vi "DFD IIR Notch Peak Design by BW.vi"(6 "fs [Hz]":dbl=1.0 format="%.2f", 7 "filter type":enum16{"Notch", "Peak"}(ring), 8 "error in (no error)":errorcluster, 9 "Ab [dB]":dbl=3.010299956639812 format="%#.6g", 10 "Df [Hz]":dbl=0.02 format="%.2f", 11 "f0 [Hz]":dbl=0.1 format="%.2f") -> (0 "error out":errorcluster, 3 "filter out":T1={"mSRate_Fs"=1.0, "mSRate_Version"="2.0", "mSRate_Comments"="", "mSRate_OrgCoef"={"type"=enum."Undefined", "gain"=1.0, "coef a (k)"=[], "coef b (v)"=[]}, "mSRate_CurCoef"={"type"=enum."Undefined", "gain"=1.0, "coef a (k)"=[], "coef b (v)"=[]}, "mSRate_Quantized?"=FALSE, "mSRate_QCoef"={"type"=enum."Undefined", "gain"=1.0, "coef a (k)"=[], "coef b (v)"=[]}, "mSRate_QSettings"=[], "mSRate_Order"=0, "mSRate_Scaling"={"mSRate_ScaleByPowerOf2?"=FALSE, "mSRate_ScaleType"=enum."No Norm"}} {"mSRate_QSettings"."source" items=["Coef a/k"=0, "Coef b/v"=7, "Input"=1, "Output"=2, "Multiplicand"=3, "Product"=4, "Sum"=5, "Delay"=6, "Gain"=8]})   [LabVIEW 2017, in "NI_DigFilterLicensed.lvlib"]
doc: "Designs a notch or peak filter in which the notch or peak is located at the center frequency. You must manually select the polymorphic instance you want to use."
uses:
  <vilib>/addons/Digital Filter Design/NI_DigFilterLicensed.lvlib
  <vilib>/addons/Digital Filter Design/_Objects.llb/DFD Filter Obj.ctl
  <vilib>/addons/Digital Filter Design/_Objects.llb/DFD Filter Coef.ctl
  <vilib>/addons/Digital Filter Design/_Objects.llb/DFD Filter Structure Type Selector.ctl
  <vilib>/addons/Digital Filter Design/_Objects.llb/dfd_Internal Quantization Settings.ctl
  <vilib>/addons/Digital Filter Design/_Objects.llb/dfd_Internal Quantization Srcs.ctl
  <vilib>/addons/Digital Filter Design/_Objects.llb/DFD Coef Norm Type.ctl
  <vilib>/addons/Digital Filter Design/NI_DigFilter_Design.lvlib
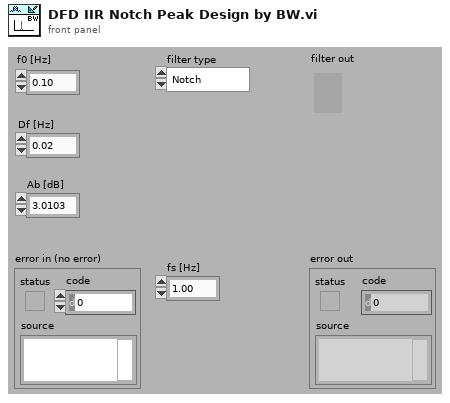
[diagram p1: front panel]
types:
  T1 = typedef "NI_DigFilterLicensed.lvlib/DFD Filter Obj.ctl" = cluster{"mSRate_Fs":dbl, "mSRate_Version":string, "mSRate_Comments":string, "mSRate_OrgCoef":T2, "mSRate_CurCoef":T2, "mSRate_Quantized?":bool, "mSRate_QCoef":T2, "mSRate_QSettings":T4[], "mSRate_Order":i32, "mSRate_Scaling":cluster{"mSRate_ScaleByPowerOf2?":bool, "mSRate_ScaleType":T6}}
  T2 = typedef "NI_DigFilterLicensed.lvlib/DFD Filter Coef.ctl" = cluster{"type":T3, "gain":dbl, "coef a (k)":dbl[], "coef b (v)":dbl[]}
  T3 = typedef "NI_DigFilterLicensed.lvlib/DFD Filter Structure Type Selector.ctl" = enum16{"Undefined", "FIR Direct Form", "FIR Direct Form Transposed", "FIR Symmetric", "FIR Antisymmetric", "IIR Direct Form I", "IIR Direct Form I Transposed", "IIR Direct Form II", "IIR Direct Form II Transposed", "IIR Cascaded Second Order Sections Form I", "IIR Cascaded Second Order Sections Form I Transposed", "IIR Cascaded Second Order Sections Form II", "IIR Cascaded Second Order Sections Form II Transposed", "Lattice Allpass (basic sections)", "Lattice Allpass (one multiplier sections)", "Lattice Allpass (normalized sections)", "Lattice AR (basic sections)", "Lattice AR (one multiplier sections)", "Lattice AR (normalized sections)", "Lattice MA (minimum phase)", "Lattice MA (maximum phase)", "Lattice ARMA (basic sections)", "Lattice ARMA (one multiplier sections)", "Lattice ARMA (normalized sections)"}
  T4 = typedef "NI_DigFilterLicensed.lvlib/dfd_Internal Quantization Settings.ctl" = cluster{"source":T5, "wl":i16, "iwl":i16, "overflow mode":enum16{"Saturation", "Wrap"}, "rounding mode":enum16{"Nearest", "Truncation"}, "signed?":bool}
  T5 = typedef "NI_DigFilterLicensed.lvlib/dfd_Internal Quantization Srcs.ctl" = u16
  T6 = typedef "NI_DigFilterLicensed.lvlib/DFD Coef Norm Type.ctl" = enum16{"No Norm", "Time Domain 1-Norm", "Time Domain 2-Norm", "Time Domain Inf-Norm"}
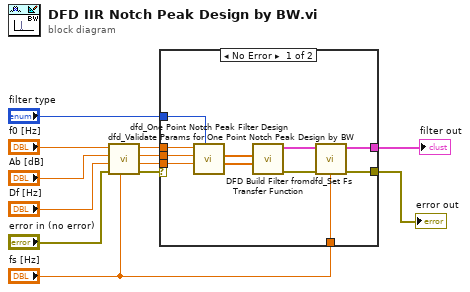
[diagram p0: block diagram]
diagram:
  n1 = call <vilib>:"dfd_Validate Params for One Point Notch Peak Design by BW.vi"("fs [Hz]"="fs [Hz]", "error in (no error)"="error in (no error)", "bandwidth"="Df [Hz]", "Ab [dB]"="Ab [dB]", "f0 [Hz]"="f0 [Hz]") -> ("error out"=w1:errorcluster, "normalized bandwidth"=w2:dbl, "dup Ab [dB]"=w3:dbl, "normalized f0"=w4:dbl)  [unwired: 3 out]
  n2 = case shown="No Error" w1 {
    selector: w1 -> [_ w24]
    tunnel: [w23 w24] -> w12
    tunnel: [w22 _] -> w11
    tunnel: "filter type" -> [w21 _]
    tunnel: w4 -> [w16 _]
    tunnel: w3 -> [w15 _]
    tunnel: w2 -> [w14 _]
    tunnel: "fs [Hz]" -> [w13 _]
    frame No Error {
      n3 = call <vilib>:"dfd_One Point Notch Peak Filter Design.vi"("filter type"=w21, "normalized BW"=w14, "Ab [dB]"=w15, "normalized f0"=w16) -> ("denominator"=w17:dbl[], "numerator"=w18:dbl[])  [unwired: 2 in, 4 out]
      n4 = call <vilib>:"DFD Build Filter from Transfer Function.vi"("denominator"=w17, "numerator"=w18) -> ("error out"=w19:errorcluster, "filter out"=w20:T1)  [unwired: 2 in, 6 out]
      n5 = call <vilib>:"dfd_Set Fs.vi"("error in (no error)"=w19, "fs [Hz]"=w13, "filter in"=w20) -> ("error out"=w23:errorcluster, "filter out"=w22:T1)  [unwired: 7 out]
    }
    frame Error {
    }
  }
  "filter out" <- w11
  "error out" <- w12
